vi "main.vi"() -> ()   [LabVIEW 2016]
panel:
  in  "start":bool
  in  "close":bool
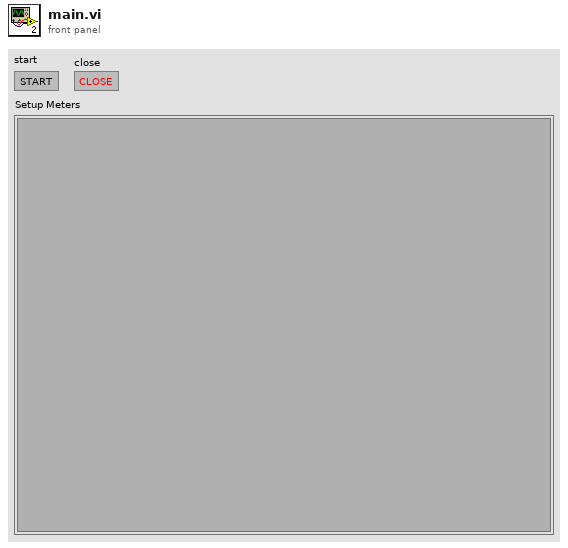
[diagram p1: front panel]
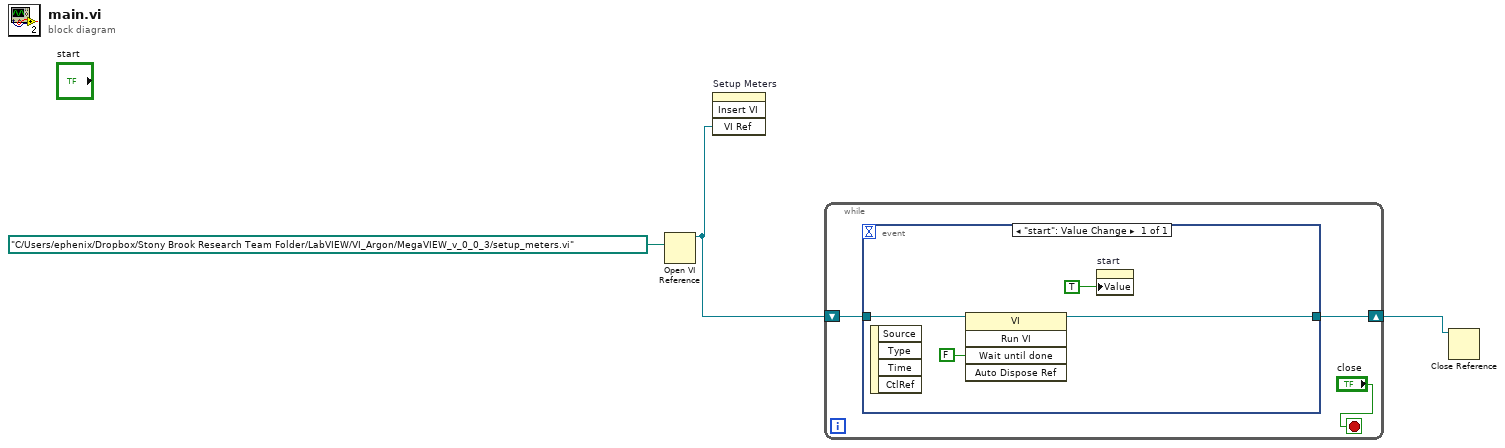
[diagram p0: block diagram]
diagram:
  n1 = Open VI Reference(vi path=path "C:/Users/ephenix/Dropbox/Stony Brook Research Team Folder/LabVIEW/VI_Argon/MegaVIEW_v_0_0_3/setup_meters.vi") -> (vi reference=w2:refnum<vi>)  [unwired: 5 in, 1 out]
  n2 = invoke on="Setup Meters" class="SubPnl" method="Insert VI"("VI Ref"=w2) -> ()  [unwired: 3 in, 4 out]
  n3 = while {
    shift-right: [w4] -> w1
    shift-left: w2 -> [w6]
    stop <- "close" stop-if-true
    n4 = event shown="[0] \"start\": Value Change" {
      selector: _ -> [_]
      dyn-events: _ -> [_]
      timeout: _ -> [_]
      tunnel: w6 -> [w9]
      tunnel: [w8] -> w4
      event "start": Value Change {
        n5 = event-data() -> ()  [unwired: 1 in, 4 out]
        n6 = invoke class="VI" method="Run VI"(reference=w9, "Wait until done"=FALSE ("Wait Until Done")) -> (reference out=w8:refnum<vi>)  [unwired: 3 in, 4 out]
        n7 = property on="start" class="Bool"("Value"=TRUE) -> ()  [unwired: 2 in, 2 out]
      }
    }
  }
  n8 = Close Reference(reference=w1) -> ()  [unwired: 1 in, 1 out]
